vi "Auto Shift.vi"(9 "Throttle":dbl, 11 "Manual Low Gear":bool) -> (3 "High Gear":bool)   [LabVIEW 2015]
uses:
  Common Code/Auto Shift State.ctl
  Robot Global Data.vi
panel:
  out "Throttle Accel":dbl
  out "Accel":dbl
  out "State":T1=enum."High"
  out "Speed":dbl
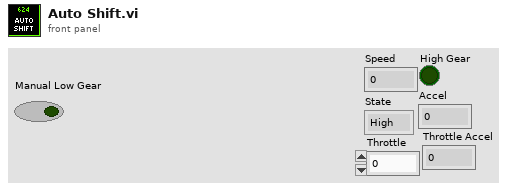
[diagram p1: front panel]
types:
  T1 = typedef "Auto Shift State.ctl" = enum16{"Low", "High"}
  T2 = typedef "Dashboard Control Data.ctl" = cluster{"Shooter Presets":T3, "Encoder Control":T5, "Steer PID output":cluster{"output high":dbl, "output low":dbl}, " Steer PID gains":cluster{"proportional gain (Kc)":dbl, "integral time (Ti, min)":dbl, "derivative time (Td, min)":dbl}, "Drivetrain Settings":T6, "Vision Packet":T7, "Dashboard Drivetrain Command":T8, "Info/Command Cluster":T10, "Ball Vision Packet":T11, "Intake Presets":T13, "Intake Encoder Control":T15, "Climb Presets":T16, "Goal Output Range":cluster{"output high":dbl, "output low":dbl}, "Enabled Systems":T17, "Auton Presets":T18, "Pressure M":dbl, "Pressure B":dbl, "Vision Timeout":dbl, "Auto-Shift":T19}
  T3 = typedef "Shooter Presets.ctl" = cluster{"Batter Shot":T4, "Deep Middle":T4, "Manual Shot":T4, "Left Ticks Per Rotation":dbl, "Right Ticks Per Rotation":dbl, "Low Bar Shot":T4, "Shooter RPM Tolerance":dbl, "Trigger Power":dbl, "Fire from Load Delay":i32, "Max Angle":dbl, "Min Angle":dbl, "Angle PID gains":cluster{"P":dbl, "I":dbl, "D":dbl}, "Angle Output":cluster{"output high":dbl, "output low":dbl}, "Shooter Angle Tolerance":dbl, "Vision Shoot x^2":dbl, "Vision Shoot x":dbl, "Feed Forward Max Accel":dbl, "Feed Forward Kv":dbl, "Backwards Trigger":dbl, "Shot Finish Delay (ms)":dbl, "Angle Max Current":dbl, "Angle Current Trip Time":dbl, "Intake Angle":dbl, "Vision Shoot c":dbl, "Reset?":bool, "Button Release Delay":dbl, "Angle Pot x":dbl, "Angle Pot c":dbl, "Ignore Angle?":bool, "Max RPM":dbl, "Safty Frist Angle":dbl, "Intake Danger Height":dbl, "Angle Pot B":i32, "Angle Pot M":dbl, "FF Finish RPM":dbl, "RPM PID Right":cluster{"P":dbl, "I":dbl, "D":dbl, "FF":dbl}, "RPM PID Left":cluster{"P":dbl, "I":dbl, "D":dbl, "FF":dbl}, "Backwards RPM":dbl, "Vision RPM":dbl, "Run Wheels Backward Delay":u32, "Cleat Shot":T4}
  T4 = typedef "Shot Presets.ctl" = cluster{"L":dbl, "R":dbl, "A":dbl}
  T5 = typedef "Encoder Control.ctl" = cluster{"Right Tick Constant":dbl, "Left Tick Constant":dbl, "Reset?":bool, "Y Dist":cluster{"PID gains":cluster{"proportional gain (Kc)":dbl, "integral time (Ti, min)":dbl, "derivative time (Td, min)":dbl}}, "Y Stop Thresh":dbl, "Y Stop Speed":dbl}
  T6 = typedef "Drivetrain Settings.ctl" = cluster{"Gyro Tolerance":dbl, "Throttle Ramp (ms)":dbl, "Kv":dbl, "Ka":dbl, "Feed Forward P":dbl, "Feed Forward D":dbl, "Goal Vision PID gains":cluster{"proportional gain (Kc)":dbl, "integral time (Ti, min)":dbl, "derivative time (Td, min)":dbl}, "Goal Detection Window":dbl, "Creep Rate":dbl, "Vision Throttle Threshold":dbl, "Min Turn Output":dbl, "Left Batter Angle":dbl, "Right Batter Angle":dbl}
  T7 = typedef "Goal Vision Packet.ctl" = cluster{"Distance":dbl, "Center X":dbl, "Center Y":dbl, "Found Target?":bool, "Robot Center":dbl, "Angle":dbl}
  T8 = typedef "Dashboard Drivetrain Command.ctl" = cluster{"Drivetrain Vision":T9}
  T9 = typedef "Drivetrain Vision.ctl" = cluster{"Goal Window":dbl, "Ball Window":dbl}
  T10 = typedef "Ball Tracking Command Cluster.ctl" = cluster{"Distance to Ball":dbl, "Desired Angle":dbl, "Command":enum16{"Turn to Ball", "Turn to Angle", "Get Distance"}, "Pixels from Center":dbl}
  T11 = typedef "Ball Vision Packet.ctl" = cluster{"Ball Detected?":bool, "Distance to Ball":dbl, "Desired Angle":dbl, "Pixels from Center":dbl, "Tracking mode":T12}
  T12 = typedef "Tracking Mode.ctl" = enum16{"Turn to Ball", "Turn to Angle"}
  T13 = typedef "Intake Presets.ctl" = cluster{"Intake Speed":dbl, "Outake Speed":dbl, "Low Height":dbl, "Half Height":dbl, "High Idle Height":dbl, "Angle Speed":dbl, "Angle Tolerance":dbl, "Encoder Scale":dbl, "Load Height":dbl, "Output Range":T14, "Rotation Power Max/Min":dbl, "MaxCurrent":dbl, "Intake Trip Time":dbl, "Idle Height":dbl, "Max Height":dbl, "Reset Encoders?":bool, "PID gains":cluster{"proportional gain (Kc)":dbl, "integral time (Ti, min)":dbl, "derivative time (Td, min)":dbl}, "Intake Stop Delay":u32, "Settle Time":dbl, "Settle Wait Time":dbl, "Pull Up Delay":dbl}
  T14 = typedef "Drivetrain Output Range.ctl" = cluster{"output high":dbl, "output low":dbl}
  T15 = typedef "IntakeEcoderControl.ctl" = cluster{"Arm Tick Constant":dbl, "Reset?":bool, "Y Dist":cluster{"PID gains":cluster{"proportional gain (Kc)":dbl, "integral time (Ti, min)":dbl, "derivative time (Td, min)":dbl}}, "Y Stop Thresh":dbl, "Y Stop Speed":dbl}
  T16 = typedef "Climb Presets.ctl" = cluster{"Pull Power":dbl, "Extend Power":dbl}
  T17 = typedef "Enabled Systems.ctl" = cluster{"Shoot":bool, "Intake":bool, "DT":bool, "Gyro":bool, "100ms":bool, "US":bool}
  T18 = typedef "Autonomous Presets.ctl" = cluster{"Pitch Limit":dbl, "Roll Limit":dbl, "Start Position":dbl, "Cross Position":dbl}
  T19 = typedef "Auto Shift Cluster.ctl" = cluster{"Delay":dbl, "Speed Thresh":dbl, "Upshift Accel":dbl, "Upshift Throttle":dbl, "Upshift Throttle Accel":dbl, "Downshift Throttle":dbl, "Downshift Throttle Accel":dbl}
  T20 = typedef "Encoder Values Super Cluster.ctl" = cluster{"Left Encoder":T21, "Right Encoder":T21}
  T21 = typedef "Encoder Values.ctl" = cluster{"Distance":dbl, "Speed":dbl, "Ticks":dbl}
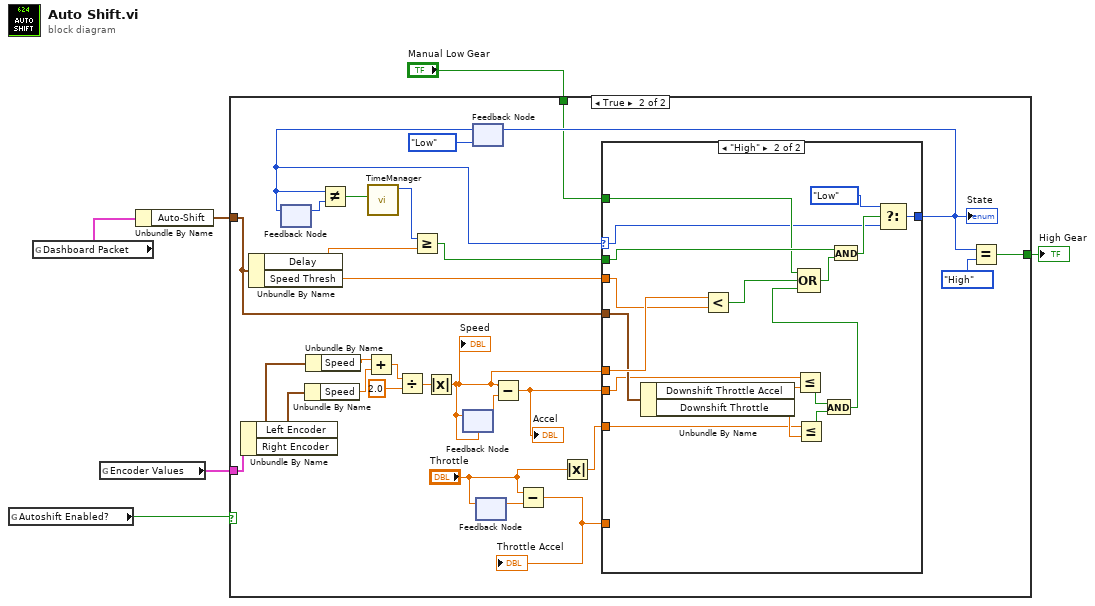
[diagram p0: block diagram]
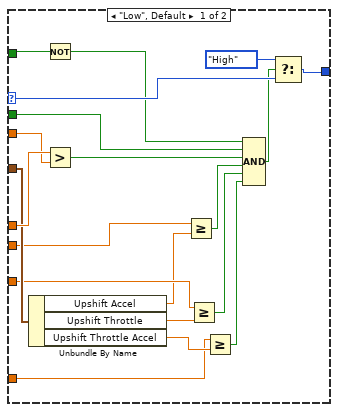
[diagram p3: hidden frame]
diagram:
  n1 = global read "Robot Global Data.vi" "Autoshift Enabled?"() -> (w1:bool)
  n2 = global read "Robot Global Data.vi" "Dashboard Packet"() -> (w6:T2)
  n3 = global read "Robot Global Data.vi" "Encoder Values"() -> (w4:T20)
  n4 = Unbundle By Name(w6) -> ("Auto-Shift"=w5:T19)
  n5 = case shown="True" w1 {
    tunnel: w5 -> [_ w12]
    tunnel: w4 -> [_ w35]
    tunnel: [w7 w18] -> w3
    tunnel: "Manual Low Gear" -> [w7 w13]
    frame False {
    }
    frame True {
      n6 = Unbundle By Name(w35) -> ("Left Encoder"=w34:T21, "Right Encoder"=w33:T21)
      n7 = Unbundle By Name(w12) -> ("Delay"=w22:dbl, "Speed Thresh"=w16:dbl)
      n8 = feedback #1() -> (w25:T1)  [unwired: 1 in]
      n9 = Unbundle By Name(w33) -> ("Speed"=w31:dbl)
      n10 = Unbundle By Name(w34) -> ("Speed"=w32:dbl)
      n11 = Add(x=w32, y=w31) -> (x+y=w30:dbl)
      n12 = Divide(x=w30, y=2.0) -> (x/y=w28:dbl)
      n13 = Absolute Value(x=w28) -> (abs(x)=w15:dbl)
      "Speed" <- w15
      n14 = feedback-in #2(w15) -> ()
      n15 = feedback #2(w15) -> (w27:dbl)
      n16 = feedback #3(Auto_Shift_State."Low") -> (w21:T1)
      n17 = feedback-in #1(w21) -> ()
      n18 = Not Equal?(x=w21, y=w25) -> (x != y?=w24:bool)
      n19 = call "TimeManager.vi"("Reset?"=w24) -> ("Time Since Reset"=w23:u32)  [unwired: 9 in, 1 out]
      n20 = Greater Or Equal?(x=w23, y=w22) -> (x >= y?=w20:bool)
      n21 = feedback #4() -> (w11:dbl)  [unwired: 1 in]
      n22 = feedback-in #4("Throttle") -> ()
      n23 = Subtract(x=w15, y=w27) -> (x-y=w14:dbl)
      "Accel" <- w14
      n24 = Subtract(x="Throttle", y=w11) -> (x-y=w8:dbl)
      "Throttle Accel" <- w8
      n25 = Absolute Value(x="Throttle") -> (abs(x)=w9:dbl)
      n26 = case shown="\"High\"" w21 {
        selector: w21 -> [w55 w69]
        tunnel: w20 -> [w50 w71]
        tunnel: [w54 w67] -> w17
        tunnel: w16 -> [w52 w64]
        tunnel: w15 -> [w53 w65]
        tunnel: w14 -> [w39 w59]
        tunnel: w13 -> [w47 w70]
        tunnel: w12 -> [w45 w63]
        tunnel: w9 -> [w41 w61]
        tunnel: w8 -> [w42 _]
        frame "Low", Default {
          n27 = Unbundle By Name(w45) -> ("Upshift Accel"=w40:dbl, "Upshift Throttle"=w44:dbl, "Upshift Throttle Accel"=w43:dbl)
          n28 = Not(x=w47) -> (.not. x?=w46:bool)
          n29 = Greater?(x=w53, y=w52) -> (0:w51:bool)
          n30 = Greater Or Equal?(x=w39, y=w40) -> (x >= y?=w38:bool)
          n31 = Greater Or Equal?(x=w41, y=w44) -> (x >= y?=w37:bool)
          n32 = Greater Or Equal?(x=w42, y=w43) -> (x >= y?=w36:bool)
          n33 = Compound Arithmetic op=AND(w46, w50, w51, w38, w37, w36) -> (w49:bool)
          n34 = Select(t=Auto_Shift_State."High", s=w49, f=w55) -> (s? t:f=w54:T1)
        }
        frame "High" {
          n35 = Unbundle By Name(w63) -> ("Downshift Throttle Accel"=w60:dbl, "Downshift Throttle"=w62:dbl)
          n36 = Less?(x=w65, y=w64) -> (x < y?=w66:bool)
          n37 = Less Or Equal?(x=w59, y=w60) -> (x <= y?=w58:bool)
          n38 = Less Or Equal?(x=w61, y=w62) -> (x <= y?=w57:bool)
          n39 = And(x=w58, y=w57) -> (x .and. y?=w56:bool)
          n40 = Compound Arithmetic op=OR(w70, w66, w56) -> (w73:bool)
          n41 = And(x=w71, y=w73) -> (x .and. y?=w72:bool)
          n42 = Select(t=Auto_Shift_State."Low", s=w72, f=w69) -> (s? t:f=w67:T1)
        }
      }
      "State" <- w17
      n43 = feedback-in #3(w17) -> ()
      n44 = Equal?(x=w17, y=Auto_Shift_State."High") -> (x = y?=w18:bool)
    }
  }
  "High Gear" <- w3
